vi "PH_Sequencer_Watch.set i attribute.vi"(0 "i ref in":refnum<vi>, 2 "i attribute":T1={"GUI Refs"={"Shot ID"=refnum, "Sequencer SM State"=refnum, "Remaining Time"=refnum, "PHELIX_Timing_T2"=refnum, "T2-Unit-Dummy"=refnum, "fs_Synchrolock_Watch"=refnum, "Experiment_Vacuum_Control_Experiment"=refnum}, "Status Synchrolock"=0, "Exp - Pressure"=0.0, "Exp - Limit"=-1.0, "Heads"=[], "Refs BooleanState"=[]} {"Status Synchrolock" items=["no info", "off/false/out", "on/true/in", "Failure", "Alarm", "Status 1", "Status 2", "Status 3"]}, 5 "error in (no error)":errorcluster) -> (14 "i ref out":refnum<vi>, 19 "error out":errorcluster)   [LabVIEW 2014, in "PH_Sequencer_Watch.lvlib"]
doc: "Sets the i attribute data of an object.\n\nLicense Agreement for this software:\n\nCopyright (C)\nGesellschaft für Schwerionenforschung, GSI\nPlanckstr. 1\n64291 Darmstadt\nGermany\n\nContact: D.Beck@gsi.de \n\nThis program is free software; you can redistribute it and/or modify it under the terms of the GNU General Public License as published by the Free Software Foundation; either version 2 of the license, or (at your option) any later version.\n\nThis program is distributed in the hope that it will be useful, but WITHOUT ANY WARRANTY; without even the implied warranty of MERCHANTABILITY or FITNESS FOR A PARTICULAR PURPOSE. See the GNU General License for more details (http://www.gnu.org).\n\nGesellschaft für Schwerionenforschung, GSI\nPlanckstr. 1, 64291 Darmstadt, Germany\nFor all questions and ideas contact: M.Richter@gsi.de, H.Brand@gsi.de or D.Beck@gsi.de.\nLast update: 17-JUN-2004"
uses:
  PH_Sequencer_Watch.lvlib
  PH_Sequencer_Watch.i attribute.ctl
  PH_Basics/PH_StatusHandler/PH_StatusHandler.Status.ctl
  PH_Sequencer_Watch.Head Information.ctl
  PH_Basics/PH_PP_Common/PH_PP_Common.PUs.ctl
  PH_Basics/PH_StatusHandler/PH_StatusHandler.lvlib
  PH_Basics/PH_PP_Common/PH_PP_Common.lvlib
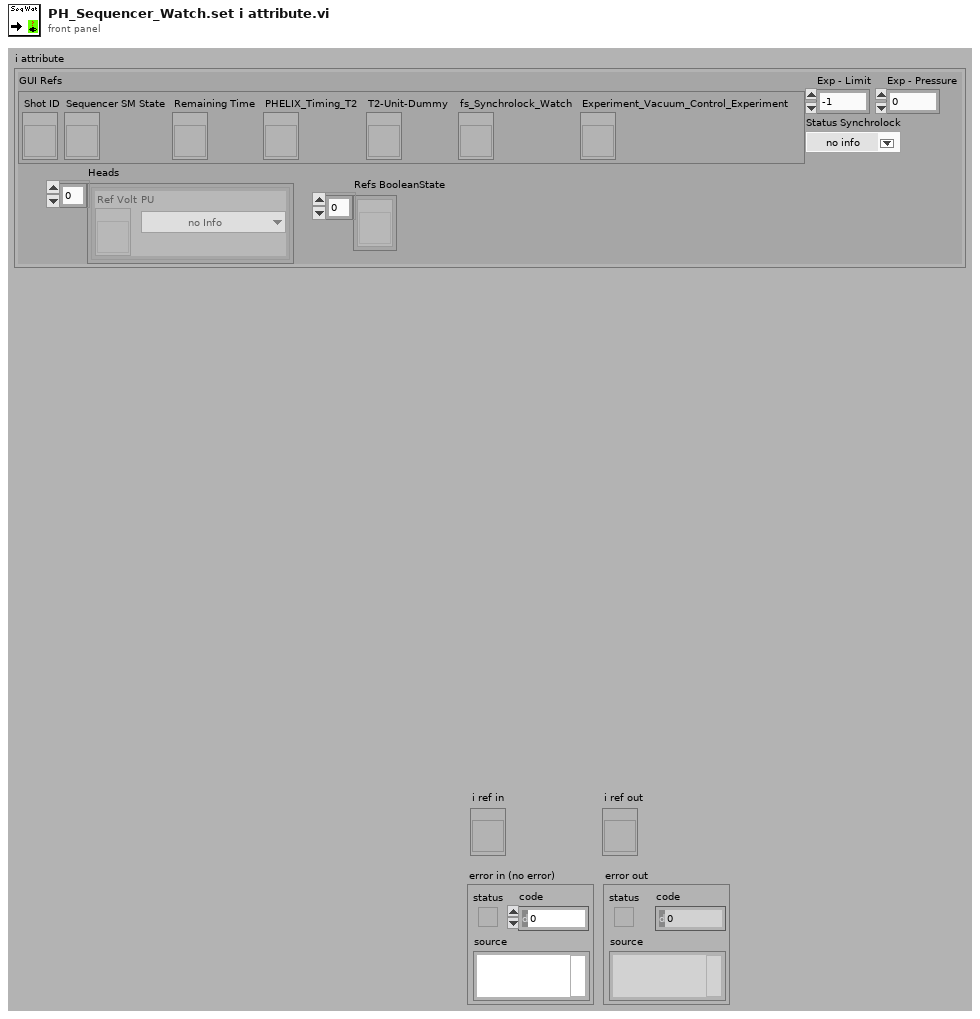
[diagram p1: front panel]
types:
  T1 = typedef "PH_Sequencer_Watch.lvlib/PH_Sequencer_Watch.i attribute.ctl" = cluster{"GUI Refs":cluster{"Shot ID":refnum<vi>, "Sequencer SM State":refnum<vi>, "Remaining Time":refnum<vi>, "PHELIX_Timing_T2":refnum<vi>, "T2-Unit-Dummy":refnum<vi>, "fs_Synchrolock_Watch":refnum<vi>, "Experiment_Vacuum_Control_Experiment":refnum<vi>}, "Status Synchrolock":T2, "Exp - Pressure":dbl, "Exp - Limit":dbl, "Heads":T3[], "Refs BooleanState":refnum<vi>[]}
  T2 = typedef "PH_StatusHandler.lvlib/PH_StatusHandler.Status.ctl" = i16
  T3 = typedef "PH_Sequencer_Watch.lvlib/PH_Sequencer_Watch.Head Information.ctl" = cluster{"Ref Volt":refnum<vi>, "PU":T4}
  T4 = typedef "PH_PP_Common.lvlib/PH_PP_Common.PUs.ctl" = enum16{"no Info", "PA-19mm-1", "PA-19mm-2", "PA-45mm-PILC", "PA-45mm-MAIN", "MA-PU-1", "MA-PU-2", "MA-PU-3", "MA-PU-4", "MA-PU-5", "MA-PU-6", "MA-FR", "MA-PILC", "PA-45mm-DP"}
  T5 = enum16{"SetAttribute", "GetAttribute", "CreateAttribute", "DestroyAttribute", "DestroyAllAtributes"}
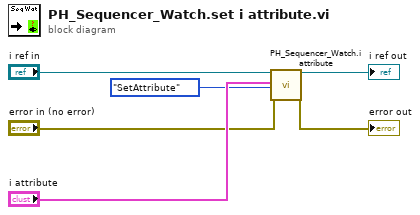
[diagram p0: block diagram]
diagram:
  n1 = call "PH_Sequencer_Watch.i attribute.vi"("VI Refnum"="i ref in", "CLASS.i attribute"="i attribute", "Action"=T5."SetAttribute", "error in (no error)"="error in (no error)") -> ("VI Refnum out"=→"i ref out":refnum<vi>, "error out"=→"error out":errorcluster)  [unwired: 13 in, 1 out]
